vi "Athena Command Main v2.vi"() -> ()   [LabVIEW 2009]
uses:
  <vilib>/userDefined/High Color/nirio_resource_hc.ctl
  <vilib>/rvi/interface/nirviOpenFPGA/nirviOpenFPGA.xnode
  FPGA Bitfiles/Athena Brain.lvproj_FPGA Target 2_FPGA Main.vi.lvbitx
  <vilib>/FPGAPlugInAG/sbRIO-9642/nirviIntfOpen_sbRIO-9642.vi
  <vilib>/rvi/interface/nirviReadWriteControl/nirviReadWriteControl.xnode
  <vilib>/Utility/error.llb/Error Cluster From Error Code.vi
  <vilib>/rvi/errors/niLvFpgaAdjustHostInterfaceError.vi
  <vilib>/rvi/interface/common/niFpgaNodeNameForErrorReporting.ctl
  <vilib>/rvi/errors/niLvFpgaWhatHappensToTopLevelVI.ctl
  UDP3-GPS, INS/UDP3GLOB.vi
  Athena Localization Data.vi
  <vilib>/LabVIEW Targets/FPGA/RIO/nirio_HostInterface/nirio_ReadBig.vi
  <vilib>/rvi/interface/nirviCloseFPGA/nirviCloseFPGA.xnode
  <vilib>/FPGAPlugInAG/sbRIO-9642/nirviIntfClose_sbRIO-9642.vi
  NiRioSrv.dll
panel:
  in  "stop":bool
  in  "Autonomus?":bool=TRUE
  in  "Steering Position Offset":i32
  in  "Steering Control Gain":fxp<+/-,20,5>=0.149993896484375 format="%.17g"
  out "Steering Enable":bool
  out "Drive Enable":bool
  out "Speed":dbl(knob) scale=0.0..10.0
  out "Meter":i32(knob) scale=-35.0..35.0
  in  "Tab Control":enum32{"Human Control", "Autonomous"}(tab)=enum."Autonomous"
  in  "Drive Enable":bool
  in  "Steering Enable":bool
  in  "Drive Speed Current (1-3.5)":fxp<+/-,18,8> format="%.13g"
  in  "Steering Position Target":i32
  out "Drive Encoder ft/sec":fxp<+/-,18,8> format="%.13g"
  in  "Wayoint":i32
  out "Drivable Paths":T1(graph)
  out "obstacle driveable path lengths":u16[](array[numeric])
  out "line driveable path lengths":u16[](array[numeric])
  in  "min obstacle dist":u16
  in  "paths to graph":enum16{"lines", "obstacles", "both"}(ring)
  in  "Auton Drive Speed Current":fxp<+/-,18,8> format="%.13g"
  in  "obstacle proximity":i16=400
  in  "line proximity":i16=100
  # "Autonomous"
  # "Human Control"
  # "-35"
  # "-30"
  # "-25"
  # "-20"
  # "-15"
  # "-10"
  # "-5"
  # "-1"
  # "1"
  # "5"
  # "10"
  # "15"
  # "20"
  # "25"
  # "30"
  # "35"
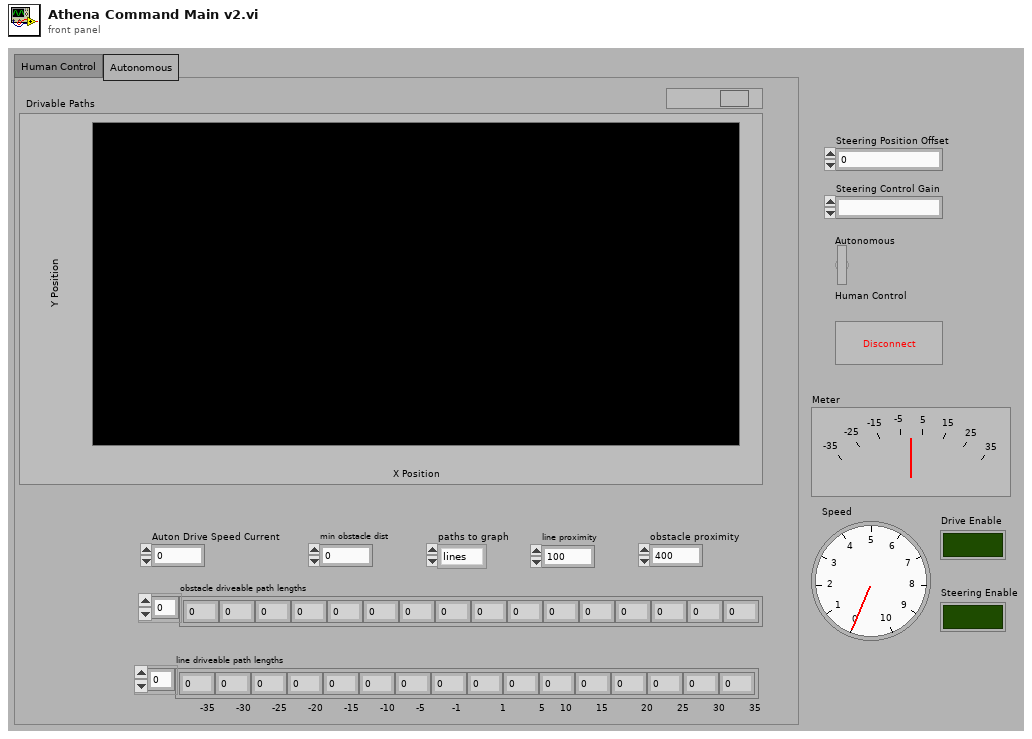
[diagram p1: front panel]
types:
  T1 = cluster{"New X Position":i16, "New Y Position":i16}[]
  T2 = typedef "nirio_resource_hc.ctl" = tag
  T3 = typedef "niFpgaNodeNameForErrorReporting.ctl" = enum16{"Open FPGA VI Reference", "Read/Write Control", "Invoke Method: Abort", "Invoke Method: Acknowledge IRQ", "Invoke Method: Download", "Invoke Method: FIFO.Configure", "Invoke Method: FIFO.Read", "Invoke Method: FIFO.Start", "Invoke Method: FIFO.Stop", "Invoke Method: FIFO.Write", "Invoke Method: Reset", "Invoke Method: Run", "Invoke Method: Wait on IRQ", "Close FPGA VI Reference"}
  T4 = typedef "niLvFpgaWhatHappensToTopLevelVI.ctl" = enum16{"top level VI scripted behind XNode", "top level VI inlined behind XNode"}
  T5 = typedef "UDP 3.ctl" = cluster{"GPS":cluster{"Lat":dbl, "Longe":dbl}, "INS":cluster{"Compass":dbl, "Altitude":dbl, "Lat":dbl, "Longe":dbl}}
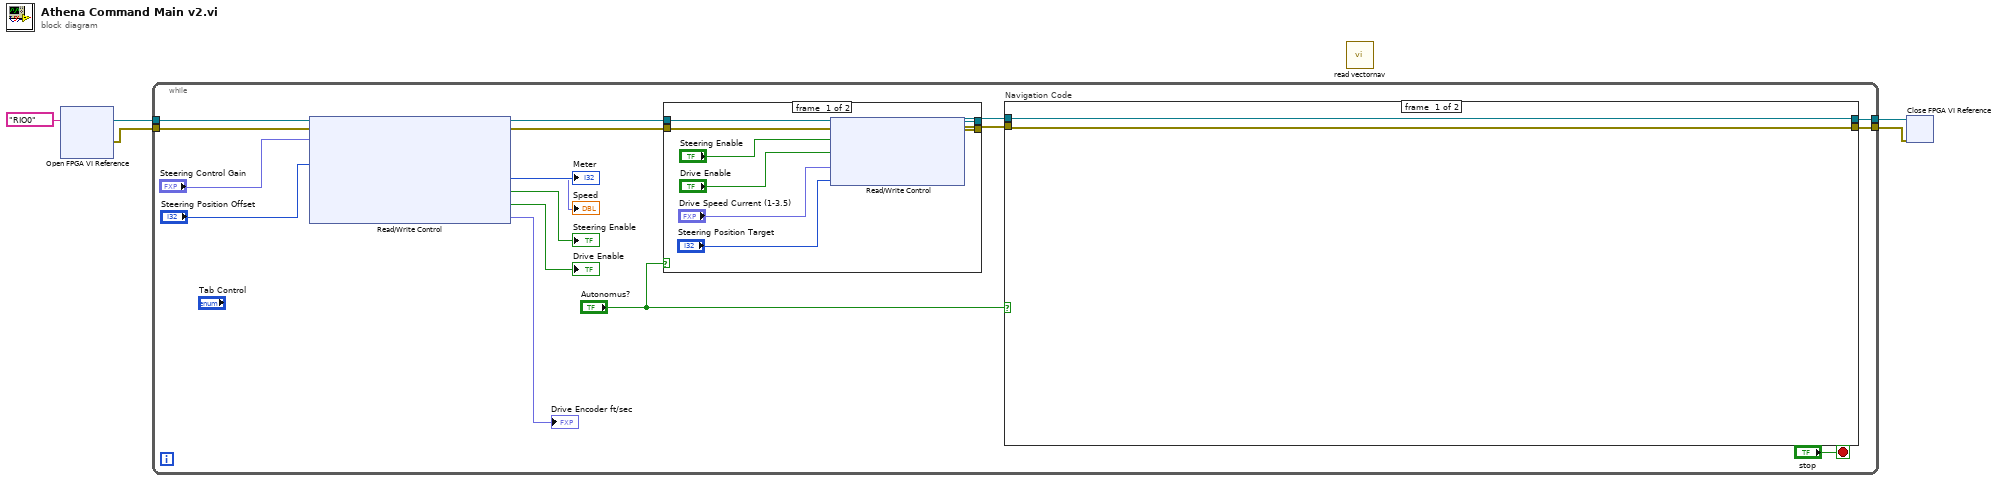
[diagram p0: block diagram]
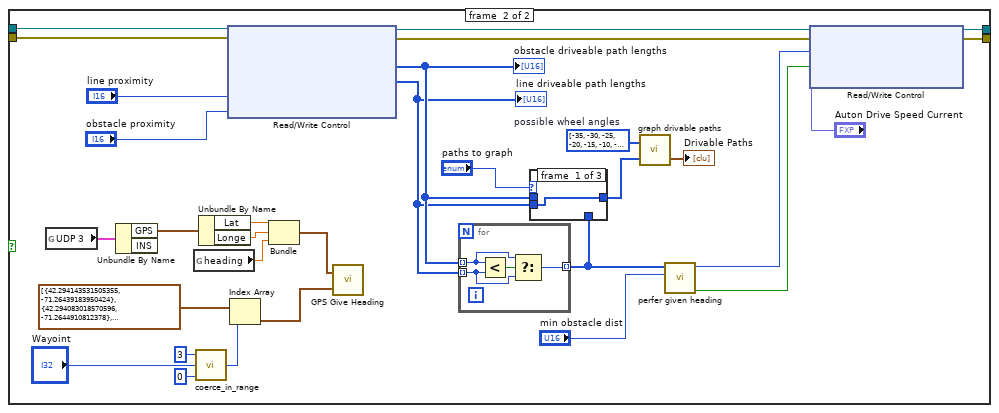
[diagram p2: hidden frame]
diagram:
  n1 = xnode "Open FPGA VI Reference"("resource name"=T2 "RIO0") -> ("FPGA VI Reference Out"=w5:refnum<k20>, "error out"=w4:errorcluster)  [unwired: 1 in]
  n2 = while {
    tunnel: w5 -> [w22]
    tunnel: w4 -> [w21]
    tunnel: [w11] -> w3
    tunnel: [w10] -> w2
    stop <- "stop" stop-if-true
    n3 = xnode "Read/Write Control"("FPGA VI Reference In"=w22, "error in"=w21, "Steering Proportional Control Feedback Gain"="Steering Control Gain", "Steering Position Offset"="Steering Position Offset") -> ("FPGA VI Reference Out"=w20:refnum<k20>, "error out"=w19:errorcluster, "Steering Position"=→"Meter":i32, "Drive Speed Current"=→"Speed":fxp<+/-,18,8>, "Steering Enabled?"=→"Steering Enable":bool, "Drive Enabled?"=→"Drive Enable":bool, "Drive Encoder ft/sec"=→"Drive Encoder ft/sec":fxp<+/-,18,8>)
    n4 = case shown="False" "Autonomus?" {
      tunnel: w20 -> [w265 w370]
      tunnel: w19 -> [w264 w369]
      tunnel: [w259 w369] -> w18
      tunnel: [w258 w370] -> w17
      frame #0 {
        n5 = xnode "Read/Write Control"("FPGA VI Reference In"=w265, "error in"=w264, "Enable Steering"="Steering Enable", "Enable Drive"="Drive Enable", "Drive Speed Current (1-3.5)"="Drive Speed Current (1-3.5)", "Steering Position Target"="Steering Position Target") -> ("FPGA VI Reference Out"=w258:refnum<k20>, "error out"=w259:errorcluster)
      }
      frame #1 {
      }
    }
    n6 = case "Navigation Code" shown="True" "Autonomus?" {
      tunnel: w18 -> [w23 w55]
      tunnel: w17 -> [w24 w54]
      tunnel: [w24 w40] -> w11
      tunnel: [w23 w41] -> w10
      frame #0 {
      }
      frame #1 {
        w53 = i8[] [-35, -30, -25, -20, -15, -10, -5, -1, 1, 5, 10, 15, 20, 25, 30, 35]  # possible wheel angles
        n7 = global read "UDP3GLOB.vi" "UDP 3"() -> (w36:T5)
        n8 = Unbundle By Name(w36) -> ("GPS"=w35:cluster{"Lat":dbl, "Longe":dbl})  [unwired: 1 out]
        n9 = global read "Athena Localization Data.vi" "heading"() -> (w32:dbl)
        n10 = call "coerce_in_range.vi"("min"=i8 0, "x"="Wayoint", "max"=i8 3) -> ("coerced x"=w25:i8)  [unwired: 2 in]
        n11 = Unbundle By Name(w35) -> ("Lat"=w34:dbl, "Longe"=w33:dbl)
        n12 = xnode "Read/Write Control"("FPGA VI Reference In"=w54, "error in"=w55, "line proximity"="line proximity", "obstacle proximity"="obstacle proximity") -> ("FPGA VI Reference Out"=w45:refnum<k20>, "error out"=w44:errorcluster, "obstacle driveable path lengths"=w48:u16[], "line driveable path lengths"=w47:u16[])  [unwired: 1 in]
        "obstacle driveable path lengths" <- w48
        "line driveable path lengths" <- w47
        n13 = Index Array(array=cluster{"Latitude":dbl, "Longitude":dbl}[] [{"Latitude"=42.294143531505355, "Longitude"=-71.26439183950424}, {"Latitude"=42.294083018570596, "Longitude"=-71.2644910812378}, {"Latitude"=42.2940443299425, "Longitude"=-71.2644575536251}, {"Latitude"=42.29408698663367, "Longitude"=-71.26439049839973}], index=w25) -> (element=w29:cluster{"Latitude":dbl, "Longitude":dbl})
        n14 = Bundle("Lat"=w34, "Longe"=w33, "heading"=w32) -> (w31:cluster{"Lat":dbl, "Longe":dbl, "heading":dbl})  [unwired: 1 in]
        n15 = call "GPS Give Heading.vi"("Target Position"=w29, "Current State"=w31) -> ()  [unwired: 2 out]
        n16 = for {
          tunnel: w48 -> [w144] mode=indexing
          tunnel: w47 -> [w143] mode=indexing
          tunnel: [w142] -> w50 mode=indexing
          n17 = Less?(x=w144, y=w143) -> (x < y?=w145:bool)
          n18 = Select(t=w144, s=w145, f=w143) -> (s? t:f=w142:u16)
        }
        n19 = case shown="\"obstacles\"" "paths to graph" {
          tunnel: w50 -> [_ _ w141]
          tunnel: w48 -> [_ w140 _]
          tunnel: w47 -> [w139 _ _]
          tunnel: [w139 w140 w141] -> w46
          frame #0 {
          }
          frame #1 {
          }
          frame #2 {
          }
        }
        n20 = call "graph drivable paths.vi"("updated max path lengths"=w46, "possible wheel angles"=w53) -> ("XY Graph"=→"Drivable Paths":T1)  [unwired: 1 in]
        n21 = call "perfer given heading.vi"("min obstacle dist"="min obstacle dist", "driveable path lengths"=w50) -> ("driveable paths?"=w42:bool, "wheel angle"=w43:i8)  [unwired: 8 in]
        n22 = xnode "Read/Write Control"("FPGA VI Reference In"=w45, "error in"=w44, "Steering Position Target"=w43, "Enable Drive"=w42, "Drive Speed Current (1-3.5)"="Auton Drive Speed Current") -> ("FPGA VI Reference Out"=w40:refnum<k20>, "error out"=w41:errorcluster)
      }
    }
  }
  n23 = call "read vectornav.vi"() -> ()  [unwired: 1 in]
  n24 = xnode "Close FPGA VI Reference"("FPGA VI Reference In"=w3, "error in"=w2) -> ()  [unwired: 1 out]
